vi "adam-build-command-analog.vi"(8 "chassis slot":u8, 9 "ADAM-5000: Chassis ID":u8=1) -> (3 "Command Out":string)   [LabVIEW 2020]
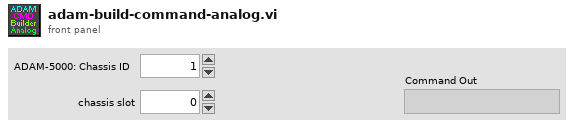
[diagram p1: front panel]
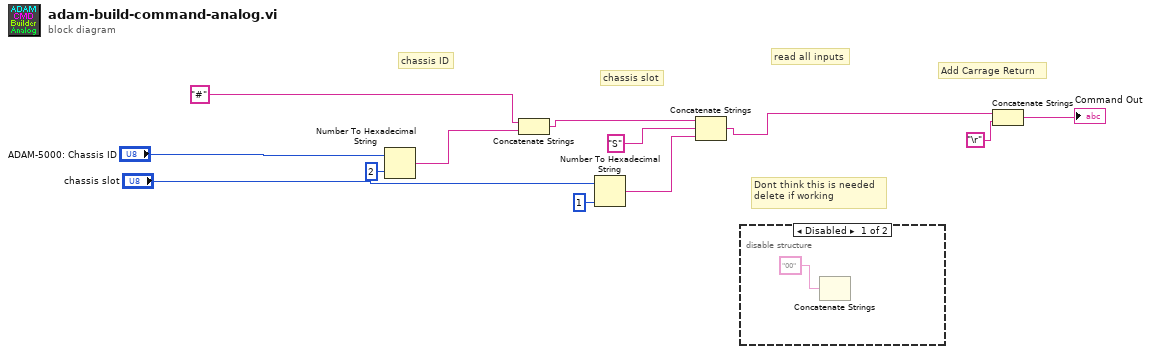
[diagram p0: block diagram]
diagram:
  # "Dont think this is needed\ndelete if working"
  # "read all inputs"
  # "Add Carrage Return"
  # "chassis slot"
  # "chassis ID"
  n1 = Number To Hexadecimal String(1:i16 2 ("width (-)"), 2:"ADAM-5000: Chassis ID") -> (0:w4:string)
  n2 = Concatenate Strings("#", w4) -> (w8:string)
  n3 = Number To Hexadecimal String(1:i16 1 ("width (-)"), 2:"chassis slot") -> (0:w10:string)
  n4 = Concatenate Strings(w8, "S" ("string"), w10) -> (w1:string)
  n5 = disable-structure shown="Disabled" {
    frame Disabled {
      n6 = Concatenate Strings("00" ("string")) -> (w14:string)  [unwired: 1 in, 1 out]
    }
    frame Enabled {
    }
  }
  n7 = Concatenate Strings(w1, "\r") -> (→"Command Out":string)
